vi "Ms to Wait with error cluster.vi"(4 "error in (no error)":errorcluster, 7 "milliseconds to wait":u32) -> (0 "error out":errorcluster, 3 "millisecond timer value":u32)   [LabVIEW 2021, in "Nanonis Prog Interface.lvlib"]
uses:
  Nanonis Prog Interface.lvlib
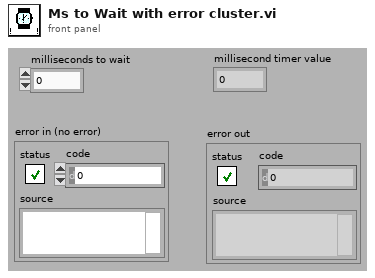
[diagram p1: front panel]
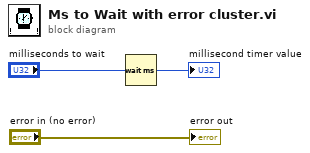
[diagram p0: block diagram]
diagram:
  n1 = Wait (ms)(milliseconds to wait="milliseconds to wait") -> (millisecond timer value=→"millisecond timer value":u32)
  "error out" <- "error in (no error)"
